vi "Single_ADC_Calc.vi"(0 "Current TH In":u32, 1 "On Delay  In":u32, 2 "SW Number Of Retry":u32, 3 "Channel OFF delay":u32, 4 "Active on startup":u8(ring) items=["Not Active", "Active"], 5 "Retry Delay In":u32, 6 "SW Retry Delay":u32, 7 "String":string, 8 "Number Of Retry In":u32, 9 "aDATA":u8[](array[numeric]), 10 "Reset Status Delay":u32, 11 "Comm. control":u8(ring) items=["Disable", "Enable"], 12 "Max curr smpl":u32, 13 "I/O control":u8(ring) items=["None", "I/O 1", "I/O 1 not", "I/O 2", "I/O 2 not", "I/O 3", "I/O 3 not ", "I/O 4", "I/O 4 not", "I/O 5", "I/O 5 not", "I/O 6", "I/O 6 not", "I/O 7", "I/O 7 not", "I/O 8 ", "I/O 8 not", "I/O 9", "I/O 9 not", "I/O 10", "I/O 10 not", "I/O 11", "I/O 11 not", "I/O 12", "I/O 12 not"]) -> (14 "Max curr smpl out":u32, 15 "I/O control out":u8(ring) items=["None", "I/O 1", "I/O 1 not", "I/O 2", "I/O 2 not", "I/O 3", "I/O 3 not ", "I/O 4", "I/O 4 not", "I/O 5", "I/O 5 not", "I/O 6", "I/O 6 not", "I/O 7", "I/O 7 not", "I/O 8 ", "I/O 8 not", "I/O 9", "I/O 9 not", "I/O 10", "I/O 10 not", "I/O 11", "I/O 11 not", "I/O 12", "I/O 12 not"], 16 "Retry Delay Out":u32, 17 "CH R":u8, 18 "SW Number Of Retry out":u32, 19 "Comm. control out":u8(ring) items=["Disable", "Enable"], 20 "Current TH Out":u32, 21 "On Delay Out":u32, 22 "Channel OFF delay out":u32, 23 "SW Retry Delay out":u32, 24 "String out":string, 25 "Number Of Retry Out":u32, 26 "Reset Status Delay out":u32, 27 "Active on startup out":u8(ring) items=["Not Active", "Active"])   [LabVIEW 2017]
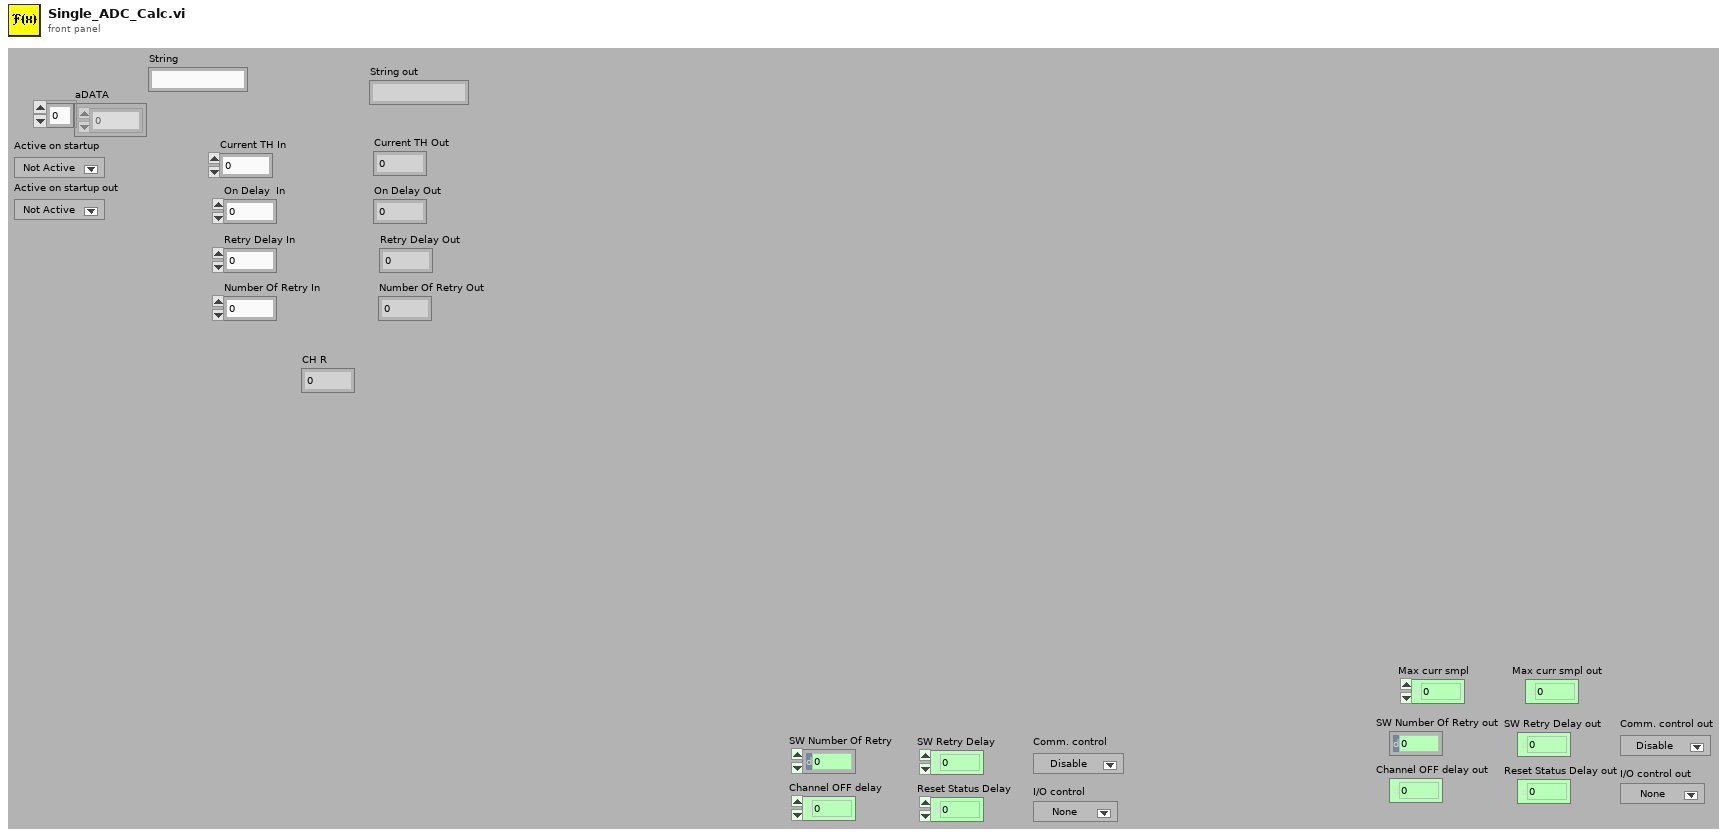
[diagram p1: front panel]
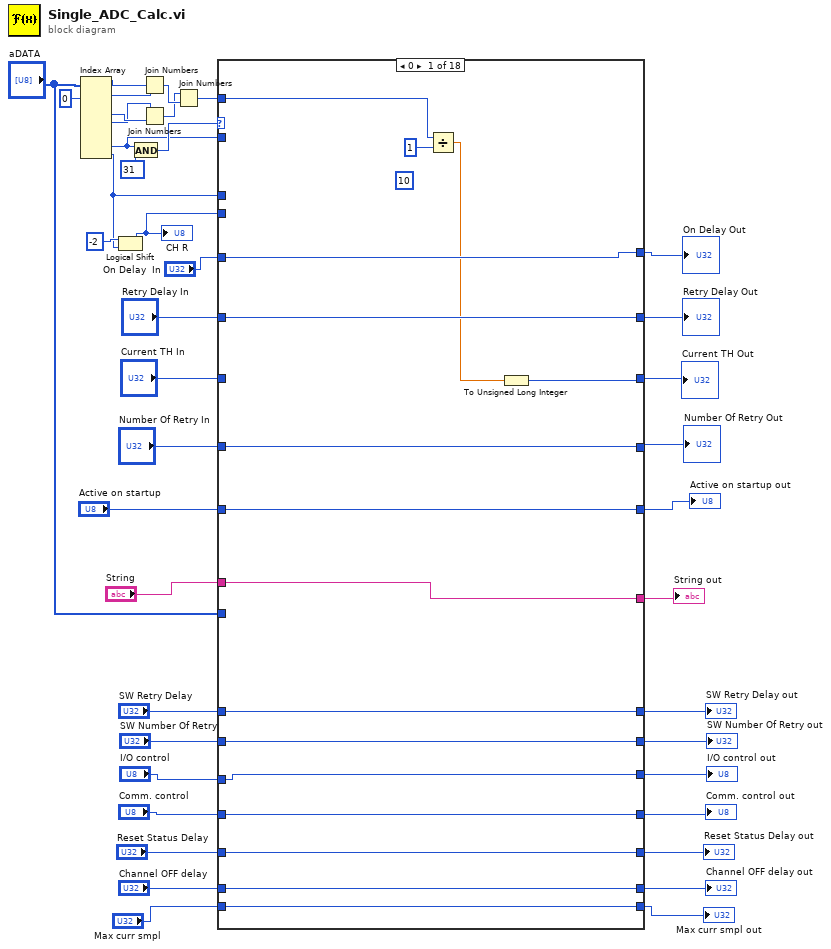
[diagram p0: block diagram]
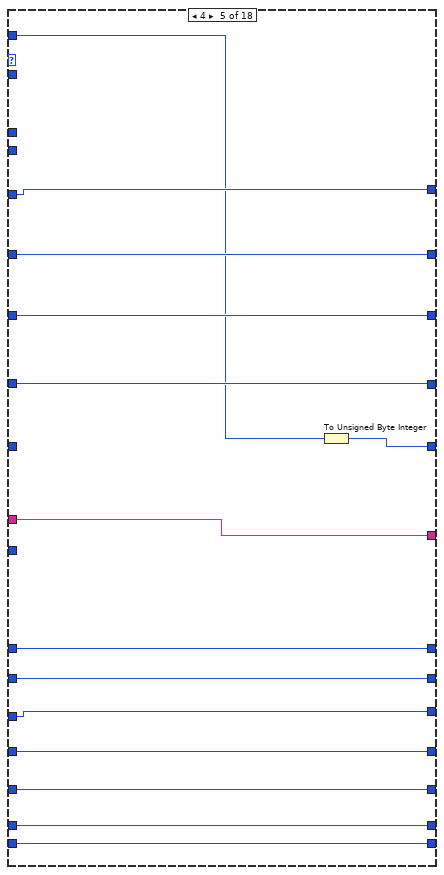
[diagram p5: hidden frame]
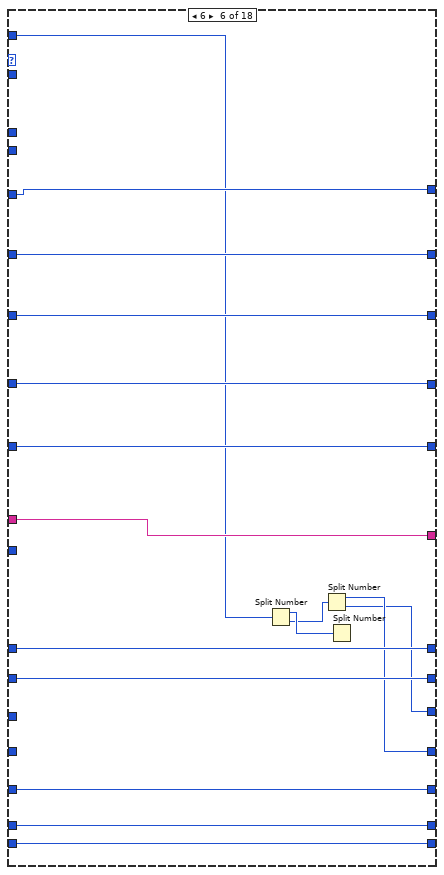
[diagram p6: hidden frame]
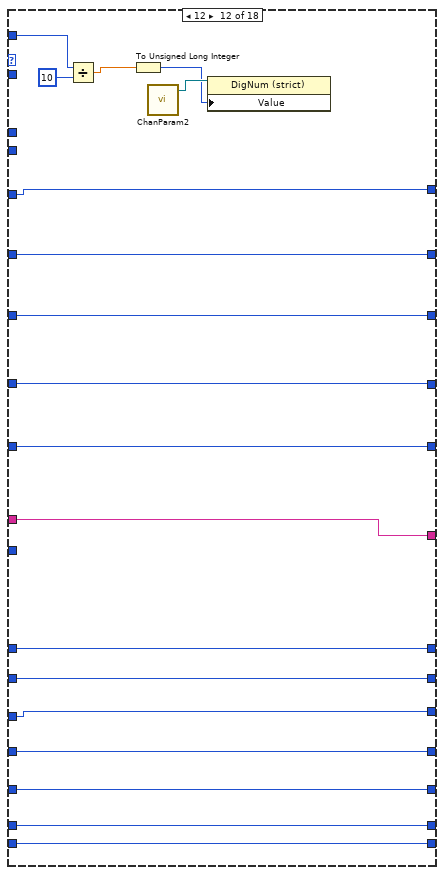
[diagram p12: hidden frame]
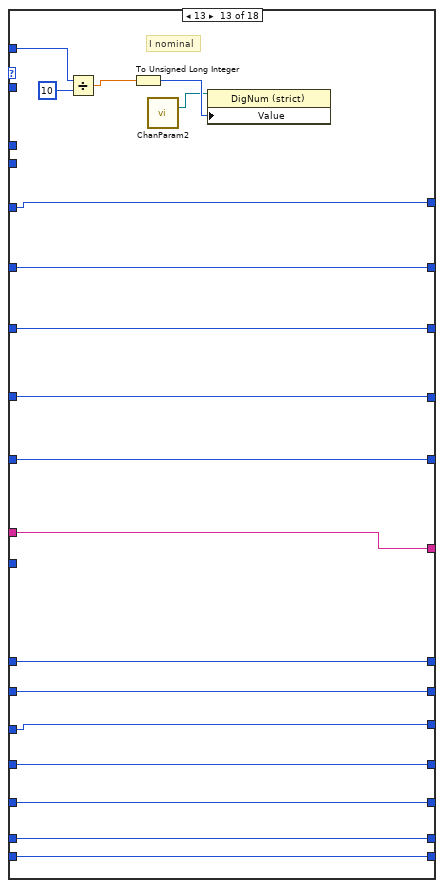
[diagram p13: hidden frame]
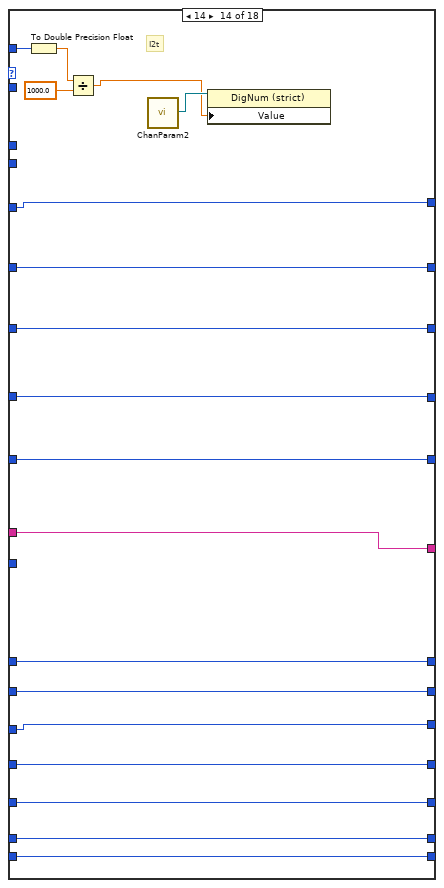
[diagram p14: hidden frame]
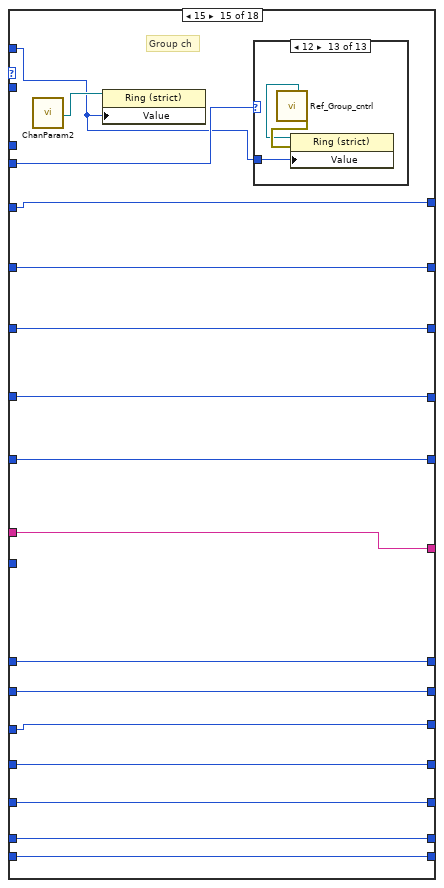
[diagram p15: hidden frame]
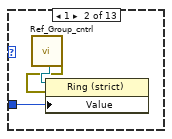
[diagram p17: hidden frame]
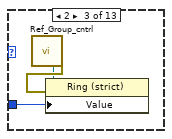
[diagram p18: hidden frame]
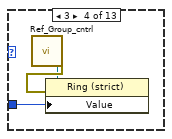
[diagram p19: hidden frame]
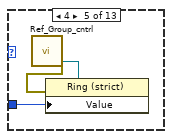
[diagram p20: hidden frame]
diagram:
  n1 = Index Array(array="aDATA", index #1=0 ("index")) -> (element #1=w36:u8, element #2=w37:u8, element #3=w39:u8, element #4=w38:u8, element #7=w16:u8, element #8=w17:u8)  [unwired: 7 in, 2 out]
  n2 = Logical Shift(y=i8 -2, x=w17) -> (x << y=w1:u8)
  "CH R" <- w1
  n3 = And(x=w16, y=u8 31) -> (x .and. y?=w20:u8)
  n4 = Join Numbers(hi=w37, lo=w36) -> ((hi.lo)=w41:u16)
  n5 = Join Numbers(hi=w38, lo=w39) -> ((hi.lo)=w40:u16)
  n6 = Join Numbers(hi=w40, lo=w41) -> ((hi.lo)=w34:u32)
  n7 = case shown="0" w20 {
    tunnel: w34 -> [w56 w70 w81 w93 w106 w118 w128 w141 w155 w168 w180 w194 w213 w231 w246 w299 _ _]
    tunnel: [w55 w70 w83 w96 w110 w126 w139 w152 w165 w178 w191 w209 w227 w245 w261 w313 w345 w358] -> w33
    tunnel: "On Delay  In" -> [w55 _ w83 w96 w110 w126 w139 w152 w165 w178 w191 w209 w227 w245 w261 w313 w345 w358]
    tunnel: "Retry Delay In" -> [w54 w68 _ w94 w108 w124 w137 w150 w163 w176 w189 w207 w225 w243 w259 w311 w343 w356]
    tunnel: [w54 w68 w81 w94 w108 w124 w137 w150 w163 w176 w189 w207 w225 w243 w259 w311 w343 w356] -> w30
    tunnel: "Current TH In" -> [_ w69 w82 w95 w109 w125 w138 w151 w164 w177 w190 w208 w226 w244 w260 w312 w344 w357]
    tunnel: [w52 w69 w82 w95 w109 w125 w138 w151 w164 w177 w190 w208 w226 w244 w260 w312 w344 w357] -> w28
    tunnel: "Number Of Retry In" -> [w51 w67 w80 _ w107 w123 w136 w149 w162 w175 w188 w206 w224 w242 w258 w310 w342 w355]
    tunnel: [w51 w67 w80 w93 w107 w123 w136 w149 w162 w175 w188 w206 w224 w242 w258 w310 w342 w355] -> w26
    tunnel: "Active on startup" -> [w50 w66 w79 w92 _ w119 w132 w145 w159 w173 w186 w204 w222 w240 w256 w308 w337 w354]
    tunnel: [w50 w66 w79 w92 w105 w119 w132 w145 w159 w173 w186 w204 w222 w240 w256 w308 w337 w354] -> w24
    tunnel: "aDATA" -> [_ _ _ _ _ _ _ _ _ _ _ _ _ _ _ _ w336 _]
    tunnel: "String" -> [w49 w65 w78 w91 w104 w122 w135 w148 w161 w174 w187 w205 w223 w241 w257 w309 w334 w353]
    tunnel: [w49 w65 w78 w91 w104 w122 w135 w148 w161 w174 w187 w205 w223 w241 w257 w309 w335 w353] -> w21
    tunnel: w17 -> [_ _ _ _ _ _ _ _ _ _ _ _ _ _ _ _ w330 _]
    tunnel: w16 -> [_ _ _ _ _ _ _ _ _ _ _ _ _ _ _ _ w333 _]
    tunnel: "SW Retry Delay" -> [w48 w64 w77 w90 w103 w115 _ w142 w156 w170 w183 w201 w219 w237 w253 w305 w324 w352]
    tunnel: "SW Number Of Retry" -> [w47 w63 w76 w89 w102 w114 w131 _ w154 w169 w182 w200 w218 w236 w252 w304 w323 w351]
    tunnel: "I/O control" -> [w46 w62 w75 w88 w101 _ w130 w144 w158 w172 w185 w203 w221 w239 w255 w307 w322 w350]
    tunnel: "Comm. control" -> [w45 w61 w74 w87 w100 _ w129 w143 w157 w171 w184 w202 w220 w238 w254 w306 w321 w349]
    tunnel: "Reset Status Delay" -> [w44 w60 w73 w86 w99 w121 w134 w147 _ w167 w181 w199 w217 w235 w251 w303 w320 w348]
    tunnel: "Channel OFF delay" -> [w43 w59 w72 w85 w98 w120 w133 w146 w160 _ w179 w198 w216 w234 w250 w302 w319 w347]
    tunnel: [w48 w64 w77 w90 w103 w115 w128 w142 w156 w170 w183 w201 w219 w237 w253 w305 w324 w352] -> w9
    tunnel: [w47 w63 w76 w89 w102 w114 w131 w141 w154 w169 w182 w200 w218 w236 w252 w304 w323 w351] -> w8
    tunnel: [w46 w62 w75 w88 w101 w112 w130 w144 w158 w172 w185 w203 w221 w239 w255 w307 w322 w350] -> w7
    tunnel: [w45 w61 w74 w87 w100 w113 w129 w143 w157 w171 w184 w202 w220 w238 w254 w306 w321 w349] -> w6
    tunnel: [w44 w60 w73 w86 w99 w121 w134 w147 w155 w167 w181 w199 w217 w235 w251 w303 w320 w348] -> w5
    tunnel: [w43 w59 w72 w85 w98 w120 w133 w146 w160 w168 w179 w198 w216 w234 w250 w302 w319 w347] -> w4
    tunnel: "Max curr smpl" -> [w42 w58 w71 w84 w97 w111 w127 w140 w153 w166 _ w197 w215 w233 w249 w301 w318 w346]
    tunnel: [w42 w58 w71 w84 w97 w111 w127 w140 w153 w166 w180 w197 w215 w233 w249 w301 w318 w346] -> w2
    tunnel: w1 -> [_ _ _ _ _ _ _ _ _ _ _ _ _ _ w247 _ _ _]
    frame 0 {
      (unwired) u32 10 ("y")
      n8 = Divide(x=w56, y=u32 1) -> (x/y=w53:dbl)
      n9 = To Unsigned Long Integer(number=w53) -> (unsigned 32bit integer=w52:u32)
    }
    frame 1 {
    }
    frame 2 {
    }
    frame 3 {
    }
    frame 4 {
      n10 = To Unsigned Byte Integer(number=w106) -> (unsigned 8bit integer=w105:u8)
    }
    frame 6 {
      n11 = Split Number(x=w118) -> (hi(x)=w117:u16, lo(x)=w116:u16)
      n12 = Split Number(x=w116) -> (hi(x)=w113:u8, lo(x)=w112:u8)
      n13 = Split Number(x=w117) -> ()  [unwired: 2 out]
    }
    frame 7 {
    }
    frame 8 {
    }
    frame 9 {
    }
    frame 10 {
    }
    frame 11 {
    }
    frame 12 {
      n14 = Divide(x=w194, y=u32 10) -> (x/y=w193:dbl)
      n15 = To Unsigned Long Integer(number=w193) -> (unsigned 32bit integer=w192:u32)
      n16 = call "ChanParam2.vi"() -> ("I Max Threshold out"=w196:refnum<vi>)  [unwired: 22 in, 5 out]
      n17 = property class="DigNum (strict)"(reference=w196, "Value"=w192) -> ()  [unwired: 1 in, 2 out]
    }
    frame 13 {
      # "I nominal"
      n18 = Divide(x=w213, y=u32 10) -> (x/y=w212:dbl)
      n19 = To Unsigned Long Integer(number=w212) -> (unsigned 32bit integer=w211:u32)
      n20 = call "ChanParam2.vi"() -> ("I Nominal out"=w210:refnum<vi>)  [unwired: 22 in, 5 out]
      n21 = property class="DigNum (strict)"(reference=w210, "Value"=w211) -> ()  [unwired: 1 in, 2 out]
    }
    frame 14 {
      # "I2t"
      n22 = To Double Precision Float(number=w231) -> (double precision float=w228:dbl)
      n23 = Divide(x=w228, y=1000.0) -> (x/y=w229:dbl)
      n24 = call "ChanParam2.vi"() -> ("I2t out"=w230:refnum<vi>)  [unwired: 22 in, 5 out]
      n25 = property class="DigNum (strict)"(reference=w230, "Value"=w229) -> ()  [unwired: 1 in, 2 out]
    }
    frame 15 {
      # "Group ch"
      n26 = call "ChanParam2.vi"() -> ("Group control out"=w248:refnum<vi>)  [unwired: 22 in, 5 out]
      n27 = property class="Ring (strict)"(reference=w248, "Value"=w246) -> ()  [unwired: 1 in, 2 out]
      n28 = case shown="12" w247 {
        tunnel: w246 -> [_ w262 w266 w269 w272 w275 w278 w281 w284 w287 w290 w293 w296]
        frame 0, Default {
        }
        frame 1 {
          n29 = call "Ref_Group_cntrl.vi"() -> ("Group ch 1 out"=w264:refnum<vi>, "error out"=w263:errorcluster)  [unwired: 15 in, 11 out]
          n30 = property class="Ring (strict)"(reference=w264, error in=w263, "Value"=w262) -> ()  [unwired: 2 out]
        }
        frame 2 {
          n31 = call "Ref_Group_cntrl.vi"() -> ("Group ch 2 out"=w265:refnum<vi>, "error out"=w267:errorcluster)  [unwired: 15 in, 11 out]
          n32 = property class="Ring (strict)"(reference=w265, error in=w267, "Value"=w266) -> ()  [unwired: 2 out]
        }
        frame 3 {
          n33 = call "Ref_Group_cntrl.vi"() -> ("Group ch 3 out"=w268:refnum<vi>, "error out"=w270:errorcluster)  [unwired: 15 in, 11 out]
          n34 = property class="Ring (strict)"(reference=w268, error in=w270, "Value"=w269) -> ()  [unwired: 2 out]
        }
        frame 4 {
          n35 = call "Ref_Group_cntrl.vi"() -> ("Group ch 4 out"=w271:refnum<vi>, "error out"=w273:errorcluster)  [unwired: 15 in, 11 out]
          n36 = property class="Ring (strict)"(reference=w271, error in=w273, "Value"=w272) -> ()  [unwired: 2 out]
        }
        frame 5 {
          n37 = call "Ref_Group_cntrl.vi"() -> ("Group ch 5 out"=w274:refnum<vi>, "error out"=w276:errorcluster)  [unwired: 15 in, 11 out]
          n38 = property class="Ring (strict)"(reference=w274, error in=w276, "Value"=w275) -> ()  [unwired: 2 out]
        }
        frame 6 {
          n39 = call "Ref_Group_cntrl.vi"() -> ("Group ch 6 out"=w277:refnum<vi>, "error out"=w279:errorcluster)  [unwired: 15 in, 11 out]
          n40 = property class="Ring (strict)"(reference=w277, error in=w279, "Value"=w278) -> ()  [unwired: 2 out]
        }
        frame 7 {
          n41 = call "Ref_Group_cntrl.vi"() -> ("Group ch 7 out"=w280:refnum<vi>, "error out"=w282:errorcluster)  [unwired: 15 in, 11 out]
          n42 = property class="Ring (strict)"(reference=w280, error in=w282, "Value"=w281) -> ()  [unwired: 2 out]
        }
        frame 8 {
          n43 = call "Ref_Group_cntrl.vi"() -> ("Group ch 8 out"=w283:refnum<vi>, "error out"=w285:errorcluster)  [unwired: 15 in, 11 out]
          n44 = property class="Ring (strict)"(reference=w283, error in=w285, "Value"=w284) -> ()  [unwired: 2 out]
        }
        frame 9 {
          n45 = call "Ref_Group_cntrl.vi"() -> ("Group ch 9 out"=w286:refnum<vi>, "error out"=w288:errorcluster)  [unwired: 15 in, 11 out]
          n46 = property class="Ring (strict)"(reference=w286, error in=w288, "Value"=w287) -> ()  [unwired: 2 out]
        }
        frame 10 {
          n47 = call "Ref_Group_cntrl.vi"() -> ("Group ch 10 out"=w289:refnum<vi>, "error out"=w291:errorcluster)  [unwired: 15 in, 11 out]
          n48 = property class="Ring (strict)"(reference=w289, error in=w291, "Value"=w290) -> ()  [unwired: 2 out]
        }
        frame 11 {
          n49 = call "Ref_Group_cntrl.vi"() -> ("Group ch 11 out"=w292:refnum<vi>, "error out"=w294:errorcluster)  [unwired: 15 in, 11 out]
          n50 = property class="Ring (strict)"(reference=w292, error in=w294, "Value"=w293) -> ()  [unwired: 2 out]
        }
        frame 12 {
          n51 = call "Ref_Group_cntrl.vi"() -> ("Group ch 12 out"=w295:refnum<vi>, "error out"=w297:errorcluster)  [unwired: 15 in, 11 out]
          n52 = property class="Ring (strict)"(reference=w295, error in=w297, "Value"=w296) -> ()  [unwired: 2 out]
        }
      }
    }
    frame 16 {
      # "techic data"
      n53 = call "ChanParam2.vi"() -> ("Tech.Data out"=w300:refnum<vi>)  [unwired: 22 in, 5 out]
      n54 = Number To Boolean Array(number=w299) -> (Boolean array=w298:bool[])
      n55 = property class="Arr (strict)"(reference=w300, "Value"=w298) -> ()  [unwired: 1 in, 2 out]
    }
    frame 5 {
      w338 = 6 ("length")
      n56 = Number To Boolean Array(number=w333) -> (Boolean array=w332:bool[])
      n57 = Number To Boolean Array(number=w330) -> (Boolean array=w328:bool[])
      n58 = Index Array(array=w328, index #1=0 ("index")) -> (element #1=w315:bool, element #2=w314:bool)  [unwired: 1 in]
      n59 = Index Array(array=w332, index #1=5 ("index")) -> (element #1=w327:bool, element #2=w317:bool, element #3=w316:bool)  [unwired: 2 in]
      n60 = Delete From Array(array=w336, length=w338, index=0) -> (deleted portion=w340:u8[])  [unwired: 1 out]
      n61 = Byte Array To String(unsigned byte array=w340) -> (string=w339:string)
      n62 = Build Array(w327, w317, w316, w315, w314) -> (w326:bool[])
      n63 = Boolean Array To Number(Boolean array=w326) -> (number=w325:u32)
      n64 = Replace Substring(2:w338, 3:w325, 4:w339, 5:w334) -> (1:w335:string)  [unwired: 1 out]
    }
    frame 100, Default {
    }
  }
  "On Delay Out" <- w33
  "Retry Delay Out" <- w30
  "Current TH Out" <- w28
  "Number Of Retry Out" <- w26
  "Active on startup out" <- w24
  "String out" <- w21
  "I/O control out" <- w7
  "Comm. control out" <- w6
  "SW Number Of Retry out" <- w8
  "SW Retry Delay out" <- w9
  "Reset Status Delay out" <- w5
  "Channel OFF delay out" <- w4
  "Max curr smpl out" <- w2
